vi "OTP - Program.vi"(2 "Save header":bool=TRUE, 3 "Max number of retries":i32=100, 4 "Read back the values written":bool, 5 "Write to device":bool, 6 "Str Refnum":refnum<vi>, 7 "Delay":u32=200, 8 "Error In":errorcluster, 9 "OTP-cal registers 2 & 3 (hex)":string[][](array[string])=[["00", "00"]], 10 "DUT info to write":T1={"Serial Number"=11, "Specification ID"="1A", "Variant"="W0", "Package"="22"}, 11 "VISA resource name":refnum<visa-resource-name>) -> (0 "error out":errorcluster)   [LabVIEW 2020]
uses:
  Devices/Controls/Device Information Cluster.ctl
  Devices/Controls/Register to Write.ctl
  Devices/PIC-device/PIC-Device.lvclass
  Devices/Device.lvclass
panel:
  in  "Stop Button":bool
  out "Return":T2
  # "REG    Action\n13     Enable VPGM to write data into the OTP ROM\n1      OTP ROM Write mode\n2     Data to Write into the OTP ROM (Upper Byte)\n3     Data to Write into the OTP ROM (Lower Byte)\n4     Address for Data Writes\n1      Back to default\n13    Back to default"
  # "REG      Action\n0           Set OTP ROM address \n5           OTP ROM Data (Upper Byte)\n6           OTP ROM Data (Lower Byte)"
  # "0x68 (104 dec) for SN\n101010101\t155\t341"
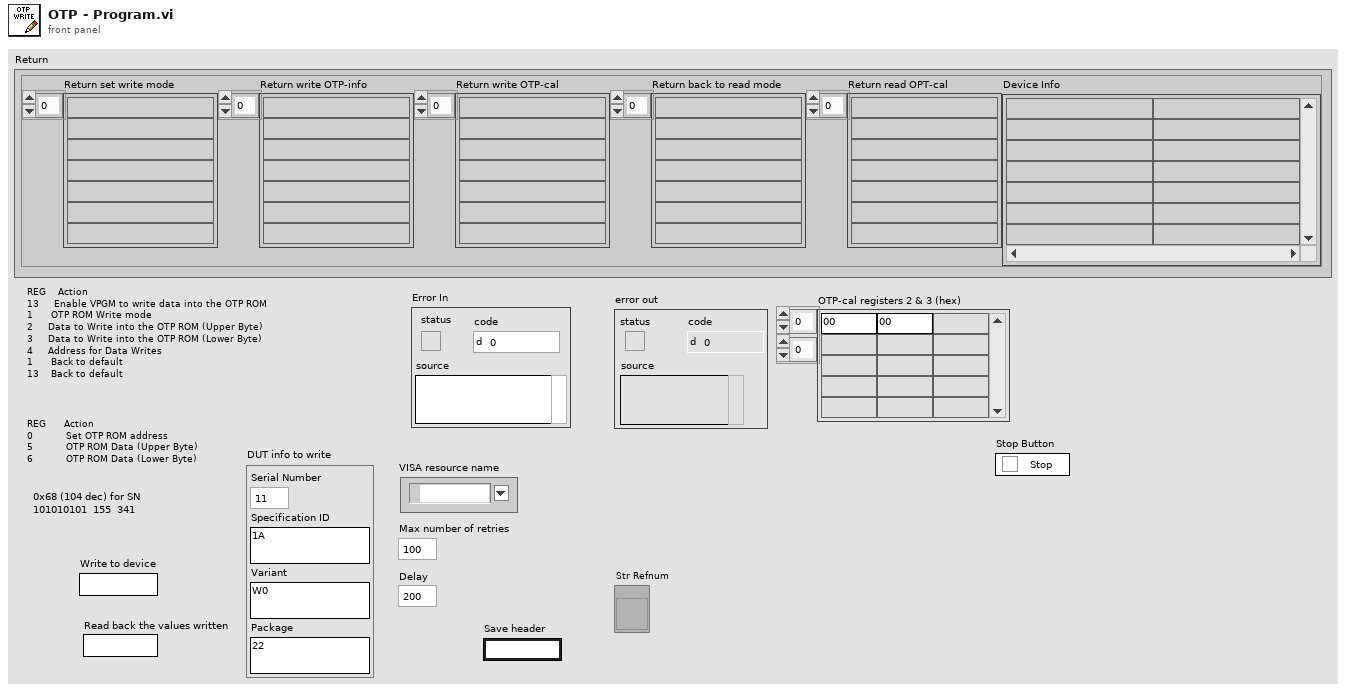
[diagram p1: front panel]
types:
  T1 = cluster{"Serial Number":u16, "Specification ID":string, "Variant":string, "Package":string}
  T2 = cluster{"Return set write mode":string[], "Return write OTP-info":string[], "Return write OTP-cal":string[], "Return back to read mode":string[], "Return read OPT-cal":string[], "Device Info":string[][]}
  T3 = typedef "PIC-Device.lvclass/Register to Write.ctl" = cluster{"Register":u32, "Value":u32, "Dev Address":u32, "Physical Adress":u32}
  T4 = typedef "Device.lvclass/Device Information Cluster.ctl" = cluster{"Device Info":string[][], "Default Values":T3[], "Fetched info":string[][]}
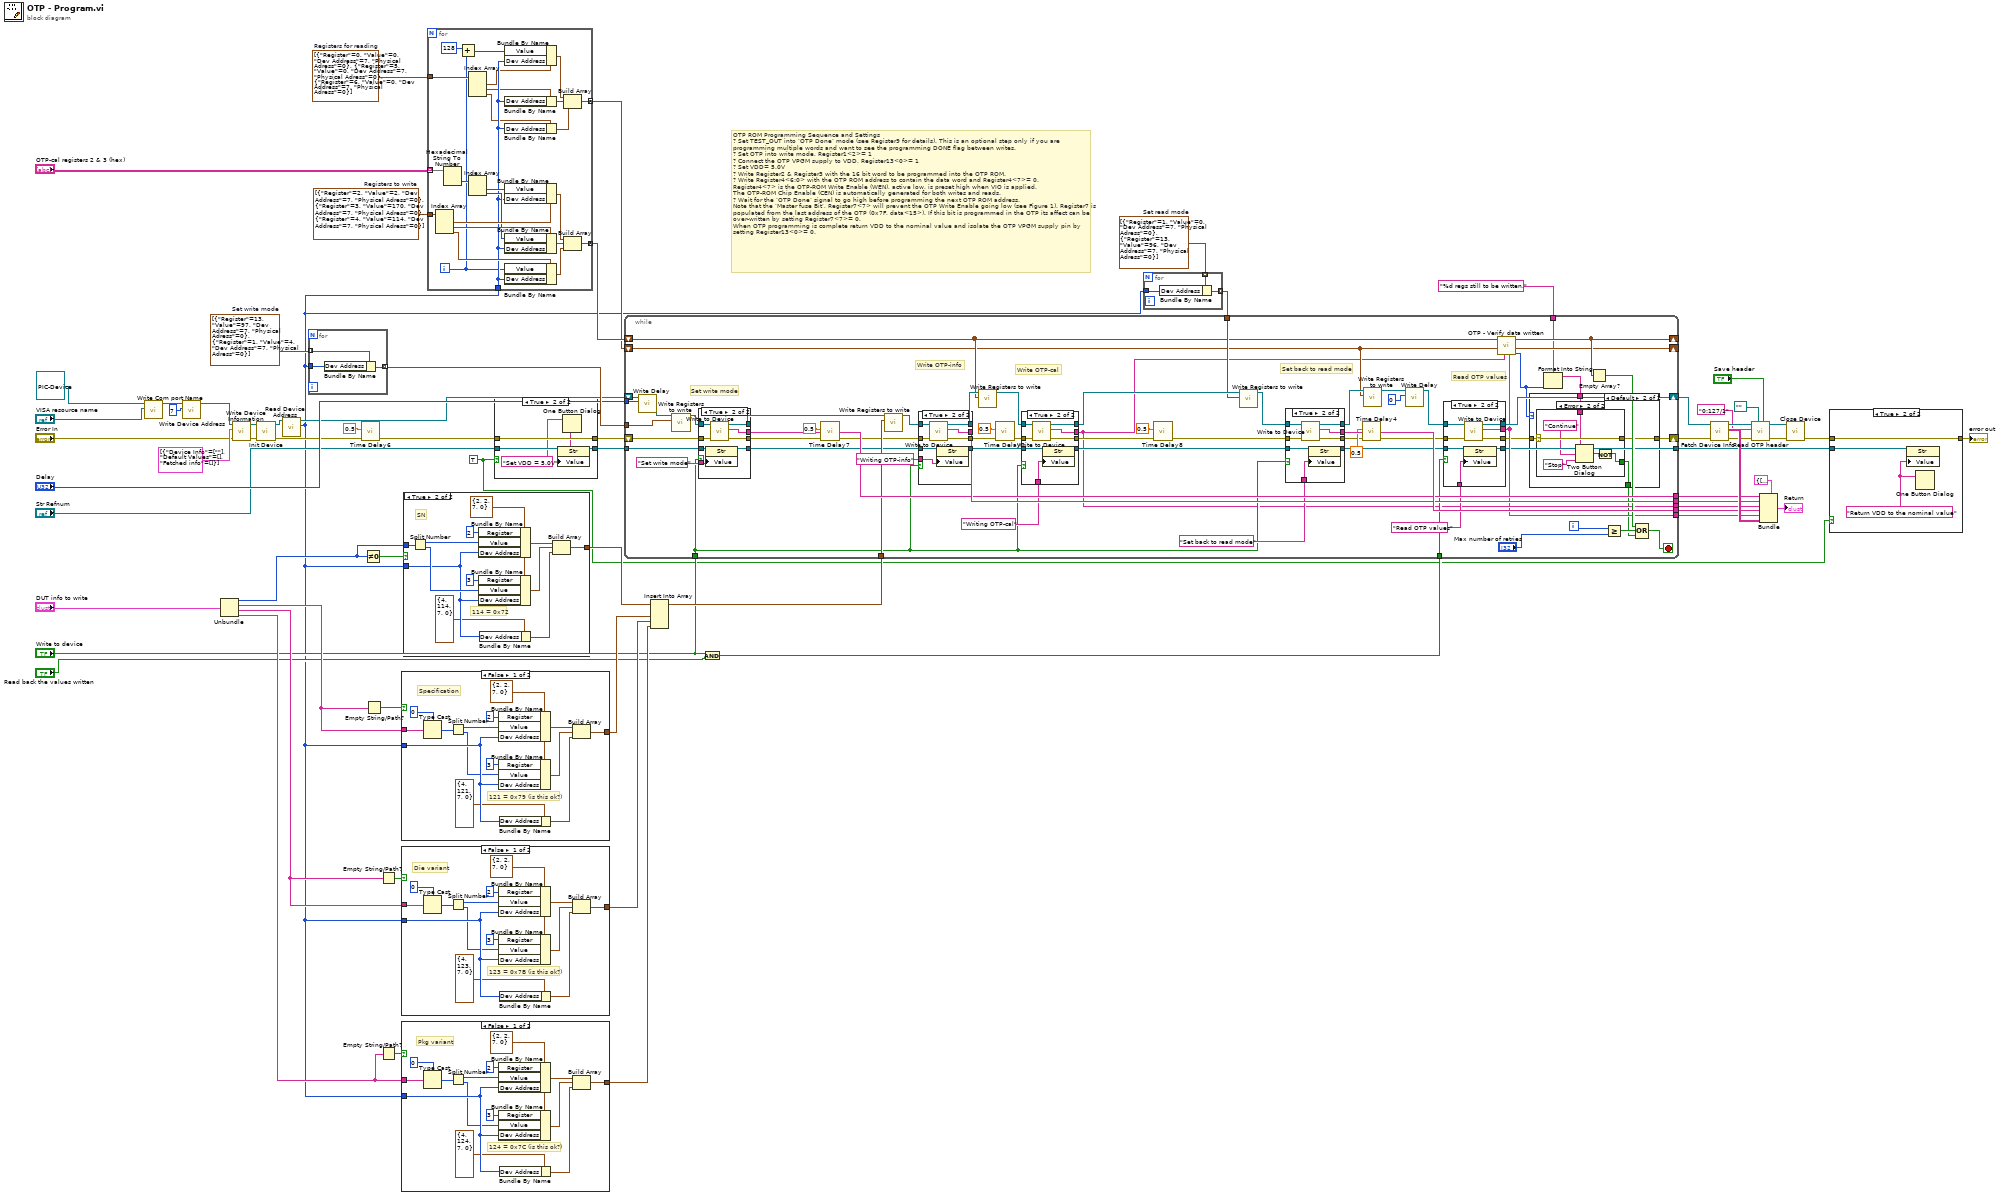
[diagram p0: block diagram]
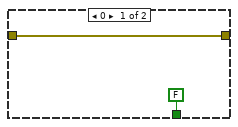
[diagram p4: hidden frame]
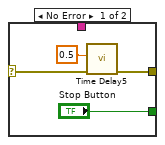
[diagram p5: hidden frame]
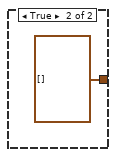
[diagram p11: hidden frame]
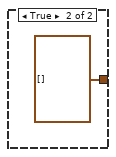
[diagram p12: hidden frame]
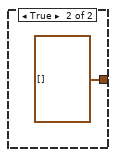
[diagram p13: hidden frame]
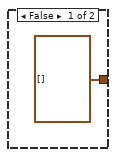
[diagram p14: hidden frame]
diagram:
  w12 = TRUE
  w54 = T3[] [{"Register"=0, "Value"=0, "Dev Address"=7, "Physical Adress"=0}, {"Register"=5, "Value"=0, "Dev Address"=7, "Physical Adress"=0}, {"Register"=6, "Value"=0, "Dev Address"=7, "Physical Adress"=0}]  # Registers for reading
  w56 = T3[] [{"Register"=2, "Value"=2, "Dev Address"=7, "Physical Adress"=0}, {"Register"=3, "Value"=170, "Dev Address"=7, "Physical Adress"=0}, {"Register"=4, "Value"=114, "Dev Address"=7, "Physical Adress"=0}]  # Registers to write
  w21 = T3[] [{"Register"=1, "Value"=0, "Dev Address"=7, "Physical Adress"=0}, {"Register"=13, "Value"=96, "Dev Address"=7, "Physical Adress"=0}]  # Set read mode
  w67 = T3[] [{"Register"=13, "Value"=97, "Dev Address"=7, "Physical Adress"=0}, {"Register"=1, "Value"=4, "Dev Address"=7, "Physical Adress"=0}]  # Set write mode
  # "OTP ROM Programming Sequence and Settings\n? Set TEST_OUT into ‘OTP Done’ mode (see Register9 for details). This is an optional step only if you are\nprogramming multiple words and want to see the programming DONE flag between writes.\n? Set OTP into write mode, Register1<2>= 1\n? Connect the OTP VPGM supply to VDD, Register13<0>= 1\n? Set VDD= 5.0V\n? Write Register2 & Register3 with the 16 bit word to be programmed into the OTP ROM.\n? Write Register4<6:0> with the OTP ROM address to contain the data word and Register4<7>= 0.\nRegister4<7> is the OTP-ROM Write Enable (WEN), active low, is preset high when VIO is applied.\nThe OTP-ROM Chip Enable (CEN) is automatically generated for both writes and reads.\n? Wait for the ‘OTP Done’ signal to go high before programming the next OTP ROM address.\nNote that the ‘Master fuse Bit’, Register7<7> will prevent the OTP Write Enable going low (see Figure 1). Register7 is\npopulated from the last address of the OTP (0x7F, data<15>). If this bit is programmed in the OTP its affect can be\nover-written by setting Register7<7>= 0.\nWhen OTP programming is complete return VDD to the nominal value and isolate the OTP VPGM supply pin by\nsetting Register13<0>= 0."
  n1 = call-dynamic "Write Com port Name.vi"("Com port Name"="VISA resource name", "Device in"=refnum<class "PIC-Device.lvclass"> refnum ("PIC-Device.lvclass")) -> ("Device out"=w64:refnum<class "PIC-Device.lvclass">)  [unwired: 9 in]
  n2 = call-dynamic "Write Device Address.vi"("Device Address"=u8 7, "PIC-Device in"=w64) -> ("PIC-Device out"=w62:refnum<class "PIC-Device.lvclass">)  [unwired: 9 in]
  n3 = Unbundle("DUT info to write") -> ("Serial Number"=w50:u16, "Specification ID"=w49:string, "Variant"=w36:string, "Package"=w38:string)
  n4 = call-dynamic "Write Device Information.vi"("error in (no error)"="Error In", "Device Info"=T4[] [{"Device Info"=[[""]], "Default Values"=[], "Fetched info"=[]}] ("Device Info 2"), "Device in"=w62) -> ("error out"=w60:errorcluster, "Device out"=w61:refnum<class "PIC-Device.lvclass">)  [unwired: 7 in]
  n5 = call-dynamic "Init Device.vi"("error in (no error)"=w60, "Device in"=w61) -> ("error out"=w28:errorcluster, "Device out"=w63:refnum<class "PIC-Device.lvclass">)  [unwired: 8 in]
  n6 = call-dynamic "Read Device Address.vi"("PIC-Device in"=w63) -> ("Device Address"=w9:u8, "PIC-Device out"=w25:refnum<class "PIC-Device.lvclass">)  [unwired: 9 in]
  n7 = for {
    tunnel: w67 -> [w70] mode=indexing
    tunnel: w9 -> [w69]
    tunnel: [w68] -> w58 mode=indexing
    n8 = Bundle By Name(cluster=w70, "Dev Address"=w69) -> (w68:T3)
  }
  n9 = call "Time Delay6"("error in (no error)"=w28, "Delay Time (s)"=0.5) -> ("error out"=w16:errorcluster)  [unwired: 9 in]
  n10 = Not Equal To 0?(x=w50) -> (x != 0?=w52:bool)
  n11 = Empty String/Path?(string/path=w49) -> (empty?=w51:bool)
  n12 = Empty String/Path?(string/path=w36) -> (empty?=w37:bool)
  n13 = Empty String/Path?(string/path=w38) -> (empty?=w39:bool)
  n14 = case shown="False" w51 {
    tunnel: w49 -> [w74 _]
    tunnel: w9 -> [w82 _]
    tunnel: [w76 T3[] []] -> w31
    frame False {
      w78 = T3 {"Register"=2, "Value"=2, "Dev Address"=7, "Physical Adress"=0} ("Register to Write")
      # "Specification"
      # "121 = 0x79 (is this ok?)"
      n15 = Type Cast(type=i16 0, x=w74) -> (*(type *) &x=w73:i16)
      n16 = Split Number(x=w73) -> (hi(x)=w72:u8, lo(x)=w71:u8)
      n17 = Bundle By Name(cluster=w78, "Register"=u32 2, "Value"=w72, "Dev Address"=w82) -> (w80:T3)
      n18 = Bundle By Name(cluster=w78, "Register"=u32 3, "Value"=w71, "Dev Address"=w82) -> (w79:T3)
      n19 = Bundle By Name(cluster=T3 {"Register"=4, "Value"=121, "Dev Address"=7, "Physical Adress"=0} ("Register to Write"), "Dev Address"=w82) -> (w77:T3)
      n20 = Build Array(w80, w79, w77) -> (w76:T3[])
    }
    frame True {
    }
  }
  n21 = case shown="False" w37 {
    tunnel: w36 -> [w89 _]
    tunnel: w9 -> [w97 _]
    tunnel: [w91 T3[] []] -> w32
    frame False {
      w93 = T3 {"Register"=2, "Value"=2, "Dev Address"=7, "Physical Adress"=0} ("Register to Write")
      # "Die variant"
      # "123 = 0x7B (is this ok?)"
      n22 = Type Cast(type=i16 0, x=w89) -> (*(type *) &x=w88:i16)
      n23 = Split Number(x=w88) -> (hi(x)=w87:u8, lo(x)=w86:u8)
      n24 = Bundle By Name(cluster=w93, "Register"=u32 2, "Value"=w87, "Dev Address"=w97) -> (w95:T3)
      n25 = Bundle By Name(cluster=w93, "Register"=u32 3, "Value"=w86, "Dev Address"=w97) -> (w94:T3)
      n26 = Bundle By Name(cluster=T3 {"Register"=4, "Value"=123, "Dev Address"=7, "Physical Adress"=0} ("Register to Write"), "Dev Address"=w97) -> (w92:T3)
      n27 = Build Array(w95, w94, w92) -> (w91:T3[])
    }
    frame True {
    }
  }
  n28 = case shown="False" w39 {
    tunnel: w38 -> [w104 _]
    tunnel: w9 -> [w112 _]
    tunnel: [w106 T3[] []] -> w33
    frame False {
      w108 = T3 {"Register"=2, "Value"=2, "Dev Address"=7, "Physical Adress"=0} ("Register to Write")
      # "Pkg variant"
      # "124 = 0x7C (is this ok?)"
      n29 = Type Cast(type=i16 0, x=w104) -> (*(type *) &x=w103:i16)
      n30 = Split Number(x=w103) -> (hi(x)=w102:u8, lo(x)=w101:u8)
      n31 = Bundle By Name(cluster=w108, "Register"=u32 2, "Value"=w102, "Dev Address"=w112) -> (w110:T3)
      n32 = Bundle By Name(cluster=w108, "Register"=u32 3, "Value"=w101, "Dev Address"=w112) -> (w109:T3)
      n33 = Bundle By Name(cluster=T3 {"Register"=4, "Value"=124, "Dev Address"=7, "Physical Adress"=0} ("Register to Write"), "Dev Address"=w112) -> (w107:T3)
      n34 = Build Array(w110, w109, w107) -> (w106:T3[])
    }
    frame True {
    }
  }
  n35 = case shown="True" w52 {
    tunnel: w50 -> [_ w128]
    tunnel: w9 -> [_ w123]
    tunnel: [T3[] [] w117] -> w35
    frame False {
    }
    frame True {
      w119 = T3 {"Register"=2, "Value"=2, "Dev Address"=7, "Physical Adress"=0} ("Register to Write")
      # "SN"
      # "114 = 0x72"
      n36 = Split Number(x=w128) -> (hi(x)=w126:u8, lo(x)=w124:u8)
      n37 = Bundle By Name(cluster=w119, "Register"=u32 2, "Value"=w126, "Dev Address"=w123) -> (w121:T3)
      n38 = Bundle By Name(cluster=w119, "Register"=u32 3, "Value"=w124, "Dev Address"=w123) -> (w120:T3)
      n39 = Bundle By Name(cluster=T3 {"Register"=4, "Value"=114, "Dev Address"=7, "Physical Adress"=0} ("Register to Write"), "Dev Address"=w123) -> (w118:T3)
      n40 = Build Array(w121, w120, w118) -> (w117:T3[])
    }
  }
  n41 = for {
    tunnel: "OTP-cal registers 2 & 3 (hex)" -> [w152] mode=indexing
    tunnel: w56 -> [w150]
    tunnel: [w141] -> w55 mode=concatenating
    tunnel: w9 -> [w136]
    tunnel: w54 -> [w140]
    tunnel: [w132] -> w53 mode=concatenating
    i -> [w134]
    n42 = Index Array(array=w150) -> (element #1=w149:T3, element #2=w147:T3, element #3=w145:T3)  [unwired: 3 in]
    n43 = Hexadecimal String To Number(string=w152) -> (number=w151:u32[])  [unwired: 2 in, 1 out]
    n44 = Add(x=u32 128, y=w134) -> (x+y=w133:u32)
    n45 = Index Array(array=w140) -> (element #1=w131:T3, element #2=w129:T3, element #3=w130:T3)  [unwired: 3 in]
    n46 = Index Array(array=w151) -> (element #1=w148:u32, element #2=w146:u32)  [unwired: 2 in]
    n47 = Bundle By Name(cluster=w131, "Value"=w133, "Dev Address"=w136) -> (w139:T3)
    n48 = Bundle By Name(cluster=w129, "Dev Address"=w136) -> (w138:T3)
    n49 = Bundle By Name(cluster=w130, "Dev Address"=w136) -> (w137:T3)
    n50 = Bundle By Name(cluster=w149, "Value"=w148, "Dev Address"=w136) -> (w144:T3)
    n51 = Bundle By Name(cluster=w147, "Value"=w146, "Dev Address"=w136) -> (w143:T3)
    n52 = Bundle By Name(cluster=w145, "Value"=w134, "Dev Address"=w136) -> (w142:T3)
    n53 = Build Array(w139, w138, w137) -> (w132:T3[])
    n54 = Build Array(w144, w143, w142) -> (w141:T3[])
  }
  n55 = case shown="True" w12 {
    tunnel: [w154 w158] -> w15
    tunnel: w16 -> [w154 w158]
    tunnel: "Str Refnum" -> [w153 w157]
    tunnel: [w153 w156] -> w13
    frame False {
    }
    frame True {
      w155 = "Set VDD = 5.0V" ("Value")
      n56 = property class="Str"(reference=w157, "Value"=w155) -> (reference out=w156:refnum<vi>)  [unwired: 1 in, 1 out]
      n57 = One Button Dialog(message=w155) -> ()  [unwired: 1 in, 1 out]
    }
  }
  n58 = Insert Into Array(array=w35, new element #1=w31, new element #2=w32, new element #3=w33) -> (w34:T3[])  [unwired: 1 in]
  n59 = And(x="Write to device", y="Read back the values written") -> (x .and. y?=w27:bool)
  n60 = for {
    tunnel: w21 -> [w161] mode=indexing
    tunnel: w9 -> [w160]
    tunnel: [w159] -> w20 mode=indexing
    n61 = Bundle By Name(cluster=w161, "Dev Address"=w160) -> (w159:T3)
  }
  n62 = while {
    tunnel: w58 -> [w224]
    tunnel: "Delay" -> [w223]
    tunnel: [w170] -> w45
    tunnel: [w215] -> w44
    tunnel: [w171] -> w43
    tunnel: [w214] -> w42
    tunnel: [w213] -> w41
    tunnel: w13 -> [w212]
    tunnel: w34 -> [w204]
    tunnel: w27 -> [w191]
    tunnel: "Write to device" -> [w188]
    shift-right: [w193] -> w30
    shift-left: w15 -> [w192]
    shift-right: [w182] -> w22
    shift-left: w25 -> [w190]
    tunnel: w20 -> [w177]
    shift-right: [w173] -> _
    shift-left: w53 -> [w172]
    shift-right: [w175] -> _
    shift-left: w55 -> [w176]
    tunnel: [w167] -> w17
    tunnel: "%d regs still to be written." ("message") -> [w165]
    i -> [w180]
    stop <- w178 stop-if-true
    # "Write OTP-info"
    # "Read OTP values"
    # "Set back to read mode"
    # "Write OTP-cal"
    # "Set write mode"
    n63 = call-dynamic "Write Delay.vi"("Delay"=w223, "PIC-Device in"=w190) -> ("PIC-Device out"=w189:refnum<class "PIC-Device.lvclass">)  [unwired: 9 in]
    n64 = call-dynamic "Write Registers to write.vi"("Registers to write"=w224, "Device in"=w189) -> ("Device out"=w225:refnum<class "PIC-Device.lvclass">)  [unwired: 9 in]
    n65 = case shown="True" w188 {
      tunnel: w225 -> [w287 w296]
      tunnel: w192 -> [w288 w295]
      tunnel: [_ w294] -> w213
      tunnel: [w287 w293] -> w217
      tunnel: [w288 w292] -> w202
      tunnel: w212 -> [w286 w291]
      tunnel: "Set write mode" -> [_ w290]
      tunnel: [w286 w289] -> w186
      frame False {
      }
      frame True {
        n66 = property class="Str"(reference=w291, "Value"=w290) -> (reference out=w289:refnum<vi>)  [unwired: 1 in, 1 out]
        n67 = call-dynamic "Write to Device.vi"("error in (no error)"=w295, "Device in"=w296) -> ("error out"=w292:errorcluster, "Return"=w294:string[], "Device out"=w293:refnum<class "PIC-Device.lvclass">)  [unwired: 7 in]
      }
    }
    n68 = call "Time Delay7"("error in (no error)"=w202, "Delay Time (s)"=0.5) -> ("error out"=w203:errorcluster)  [unwired: 9 in]
    n69 = call-dynamic "Write Registers to write.vi"("Registers to write"=w204, "Device in"=w217) -> ("Device out"=w218:refnum<class "PIC-Device.lvclass">)  [unwired: 9 in]
    n70 = case shown="True" w188 {
      tunnel: [_ w252] -> w214
      tunnel: [w243 w251] -> w195
      tunnel: w203 -> [w243 w250]
      tunnel: w218 -> [w244 w249]
      tunnel: [w244 w248] -> w216
      tunnel: "Writing OTP-info" -> [_ w247]
      tunnel: w186 -> [w242 w246]
      tunnel: [w242 w245] -> w206
      frame False {
      }
      frame True {
        n71 = call-dynamic "Write to Device.vi"("error in (no error)"=w250, "Device in"=w249) -> ("error out"=w251:errorcluster, "Return"=w252:string[], "Device out"=w248:refnum<class "PIC-Device.lvclass">)  [unwired: 7 in]
        n72 = property class="Str"(reference=w246, "Value"=w247) -> (reference out=w245:refnum<vi>)  [unwired: 1 in, 1 out]
      }
    }
    n73 = call-dynamic "Write Registers to write.vi"("Registers to write"=w176, "Device in"=w216) -> ("Device out"=w221:refnum<class "PIC-Device.lvclass">)  [unwired: 9 in]
    n74 = call "Time Delay2"("error in (no error)"=w195, "Delay Time (s)"=0.5) -> ("error out"=w194:errorcluster)  [unwired: 9 in]
    n75 = case shown="True" w188 {
      tunnel: [_ w285] -> w171
      tunnel: [w276 w284] -> w196
      tunnel: w194 -> [w276 w283]
      tunnel: w221 -> [w277 w282]
      tunnel: [w277 w281] -> w219
      tunnel: "Writing OTP-cal" -> [_ w280]
      tunnel: w206 -> [w275 w279]
      tunnel: [w275 w278] -> w183
      frame False {
      }
      frame True {
        n76 = call-dynamic "Write to Device.vi"("error in (no error)"=w283, "Device in"=w282) -> ("error out"=w284:errorcluster, "Return"=w285:string[], "Device out"=w281:refnum<class "PIC-Device.lvclass">)  [unwired: 7 in]
        n77 = property class="Str"(reference=w279, "Value"=w280) -> (reference out=w278:refnum<vi>)  [unwired: 1 in, 1 out]
      }
    }
    n78 = call "Time Delay8"("error in (no error)"=w196, "Delay Time (s)"=0.5) -> ("error out"=w197:errorcluster)  [unwired: 9 in]
    n79 = call-dynamic "Write Registers to write.vi"("Registers to write"=w177, "Device in"=w219) -> ("Device out"=w220:refnum<class "PIC-Device.lvclass">)  [unwired: 9 in]
    n80 = case shown="True" w188 {
      tunnel: [_ w274] -> w215
      tunnel: [w265 w273] -> w222
      tunnel: [w266 w270] -> w198
      tunnel: w197 -> [w266 w272]
      tunnel: w220 -> [w265 w271]
      tunnel: "Set back to read mode" -> [_ w269]
      tunnel: w183 -> [w264 w268]
      tunnel: [w264 w267] -> w205
      frame False {
      }
      frame True {
        n81 = call-dynamic "Write to Device.vi"("error in (no error)"=w272, "Device in"=w271) -> ("error out"=w270:errorcluster, "Return"=w274:string[], "Device out"=w273:refnum<class "PIC-Device.lvclass">)  [unwired: 7 in]
        n82 = property class="Str"(reference=w268, "Value"=w269) -> (reference out=w267:refnum<vi>)  [unwired: 1 in, 1 out]
      }
    }
    n83 = call "Time Delay4"("error in (no error)"=w198, "Delay Time (s)"=0.5) -> ("error out"=w199:errorcluster)  [unwired: 9 in]
    n84 = call-dynamic "Write Registers to write.vi"("Registers to write"=w172, "Device in"=w222) -> ("Device out"=w185:refnum<class "PIC-Device.lvclass">)  [unwired: 9 in]
    n85 = call-dynamic "Write Delay.vi"("Delay"=u32 0, "PIC-Device in"=w185) -> ("PIC-Device out"=w184:refnum<class "PIC-Device.lvclass">)  [unwired: 9 in]
    n86 = case shown="True" w191 {
      tunnel: [w255 w263] -> w162
      tunnel: [w254 w262] -> w182
      tunnel: [_ w261] -> w170
      tunnel: w184 -> [w254 w260]
      tunnel: w199 -> [w255 w259]
      tunnel: "Read OTP values" -> [_ w258]
      tunnel: w205 -> [w253 w257]
      tunnel: [w253 w256] -> w167
      frame False {
      }
      frame True {
        n87 = property class="Str"(reference=w257, "Value"=w258) -> (reference out=w256:refnum<vi>)  [unwired: 1 in, 1 out]
        n88 = call-dynamic "Write to Device.vi"("error in (no error)"=w259, "Device in"=w260) -> ("error out"=w263:errorcluster, "Return"=w261:string[], "Device out"=w262:refnum<class "PIC-Device.lvclass">)  [unwired: 7 in]
      }
    }
    n89 = call "OTP - Verify data written.vi"("Read Return"=w170, "Write Return"=w171, "Read in"=w172, "write in"=w176) -> ("# of regs still to be written"=w163:i32, "Read out"=w173:T3[], "write out"=w175:T3[])  [unwired: 5 in]
    n90 = Format Into String(format string=w165, w163) -> (resulting string=w164:string)  [unwired: 2 in, 1 out]
    n91 = case shown="Default" w163 {
      tunnel: w162 -> [w227 w231]
      tunnel: [w227 w230] -> w193
      tunnel: [FALSE ("Stop Button") w229] -> w166
      tunnel: w164 -> [_ w228]
      frame 0 {
      }
      frame Default {
        n92 = case shown="Error" w231 {
          selector: w231 -> [w234 w239]
          tunnel: [w233 w239] -> w230
          tunnel: ["Stop Button" w240] -> w229
          tunnel: w228 -> [_ w238]
          frame No Error {
            n93 = call "Time Delay5"("error in (no error)"=w234, "Delay Time (s)"=0.5) -> ("error out"=w233:errorcluster)  [unwired: 9 in]
          }
          frame Error {
            n94 = Two Button Dialog(message=w238, 1:"Stop" ("F button name (\"Cancel\")"), 2:"Continue" ("T button name (\"OK\")")) -> (T button?=w241:bool)
            n95 = Not(x=w241) -> (.not. x?=w240:bool)
          }
        }
      }
    }
    n96 = Empty Array?(array=w175) -> (empty?=w174:bool)
    n97 = Greater Or Equal?(x=w180, y="Max number of retries") -> (x >= y?=w179:bool)
    n98 = Compound Arithmetic op=OR(w174, w179, w166) -> (w178:bool)
  }
  n99 = call-dynamic "Fetch Device Info.vi"("error in (no error)"=w30, "PIC-Device in"=w22) -> ("error out"=w7:errorcluster, "Device Info"=w46:string[][], "PIC-Device out"=w6:refnum<class "PIC-Device.lvclass">)  [unwired: 7 in]
  n100 = call-dynamic "Read OTP header.vi"("Write to file"="Save header", "selected path"=path "", "error in (no error)"=w7, "OTP values to read"="0:127/1", "PIC-Device in"=w6) -> ("error out"=w4:errorcluster, "PIC-Device out"=w5:refnum<class "PIC-Device.lvclass">)  [unwired: 4 in, 1 out]
  n101 = Bundle(cluster=T2 {"Return set write mode"=[], "Return write OTP-info"=[], "Return write OTP-cal"=[], "Return back to read mode"=[], "Return read OPT-cal"=[], "Device Info"=[]} ("Return"), "Return set write mode"=w41, "Return write OTP-info"=w42, "Return write OTP-cal"=w43, "Return back to read mode"=w44, "Return read OPT-cal"=w45, "Device Info"=w46) -> (→"Return":T2)
  n102 = call-dynamic "Close Device.vi"("error in (no error)"=w4, "Device in"=w5) -> ("error out"=w19:errorcluster)  [unwired: 8 in, 1 out]
  n103 = case shown="True" w12 {
    tunnel: [w297 w300] -> w18
    tunnel: w19 -> [w297 w300]
    tunnel: w17 -> [_ w299]
    frame False {
    }
    frame True {
      w298 = "Return VDD to the nominal value" ("Value")
      n104 = property class="Str"(reference=w299, "Value"=w298) -> ()  [unwired: 1 in, 2 out]
      n105 = One Button Dialog(message=w298) -> ()  [unwired: 1 in, 1 out]
    }
  }
  "error out" <- w18
